vi "Get Pos.vi"(8 "error in (no error)":errorcluster, 11 "Motor in":refnum<class "Motor.lvclass">) -> (0 "error out":errorcluster, 1 "Position in display unit (frontend)":dbl, 2 "Position in display unit (backend)":dbl, 3 "Motor out":refnum<class "Motor.lvclass">)   [LabVIEW 2016, in "Hardware.lvlib" / "Motor.lvlib" / "Motor.lvclass"]
uses:
  <userlib>/Common Components/Hardware/Motor/Motor/Motor.lvclass
  <userlib>/Common Components/Hardware/Motor/Motor/Motor.lvclass/Motor.ctl
panel:
  # "encoder pos if encoder equipped;\notherwise motor pos\n\nbackend pos used for every internal operation\nfrontend pos just for display to users"
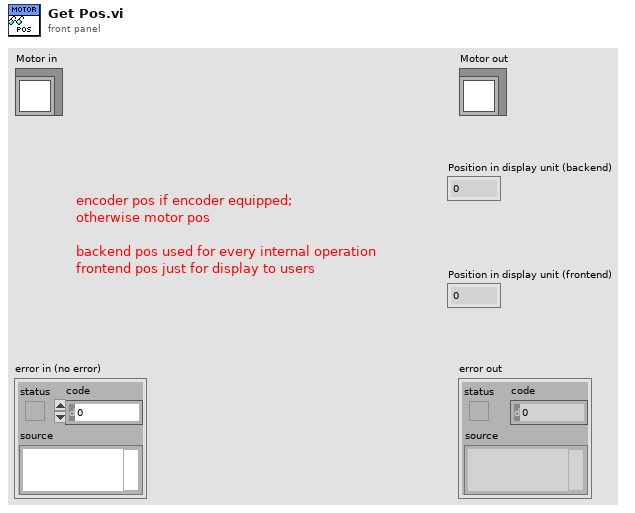
[diagram p1: front panel]
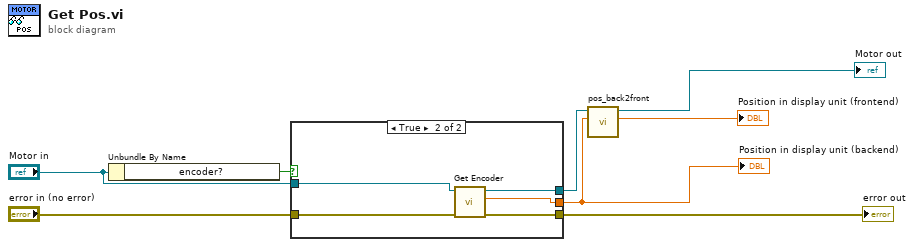
[diagram p0: block diagram]
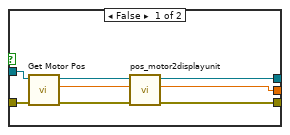
[diagram p2: hidden frame]
diagram:
  n1 = Unbundle By Name("Motor in") -> ("encoder?"=w8:bool)
  n2 = case shown="True" w8 {
    tunnel: "Motor in" -> [w16 w21]
    tunnel: "error in (no error)" -> [w15 w20]
    tunnel: [w11 w19] -> w6
    tunnel: [w9 w18] -> w4
    tunnel: [w10 w17] -> w2
    frame False {
      n3 = call-dynamic "Get Motor Pos.vi"("error in (no error)"=w15, "Motor in"=w16) -> ("error out"=w12:errorcluster, "motor pos (pulse)"=w13:dbl, "Motor out"=w14:refnum<class "Motor.lvclass">)  [unwired: 7 in]
      n4 = call <userlib>:"pos_motor2displayunit.vi"("error in (no error)"=w12, "pos in motor (pulses)"=w13, "Motor in"=w14) -> ("error out"=w9:errorcluster, "pos in display unit"=w10:dbl, "Motor out"=w11:refnum<class "Motor.lvclass">)  [unwired: 6 in]
    }
    frame True {
      n5 = call <userlib>:"Get Encoder.vi"("error in (no error)"=w20, "Motor in"=w21) -> ("error out"=w18:errorcluster, "encoder pos in display unit"=w17:dbl, "Motor out"=w19:refnum<class "Motor.lvclass">)  [unwired: 7 in]
    }
  }
  "error out" <- w4
  "Position in display unit (backend)" <- w2
  n6 = call <userlib>:"pos_back2front.vi"("pos backend"=w2, "Motor in"=w6) -> ("pos frontend"=→"Position in display unit (frontend)":dbl, "Motor out"=→"Motor out":refnum<class "Motor.lvclass">)  [unwired: 7 in, 1 out]
